vi "Module Template SM.vi"(8 "error in (no error)":errorcluster, 11 "Module_Refs":T1={"ModuleName"=enum."Controller", "Queue"=refnum, "user event"=refnum, "VI Refnum"=refnum, "ShowFP"=FALSE, "StatesTracking Enabled"=FALSE}) -> (0 "error out":errorcluster)   [LabVIEW 2021, in "Module Template.lvlib"]
doc: "Main Module Template of the architecture. Use this as a template to integrate new independent processes into your application."
uses:
  Module Template.lvlib
  Typedefs/Module References.ctl
  Typedefs/Enum_Module_Name.ctl
  Typedefs/Message.ctl
  Typedefs/State Machine Data.ctl
  Typedefs/Config.ctl
  Typedefs/Application Configuration.ctl
  Module Template Configuraton Extractor API.vi
  Configuration/Configuration.lvlib
  Architecture.lvlib
panel:
  in  "Stop App":bool
  out "Message":string
  in  "Stop Module":bool
  # "#Architecture\n\nPlace inside this box all visible data."
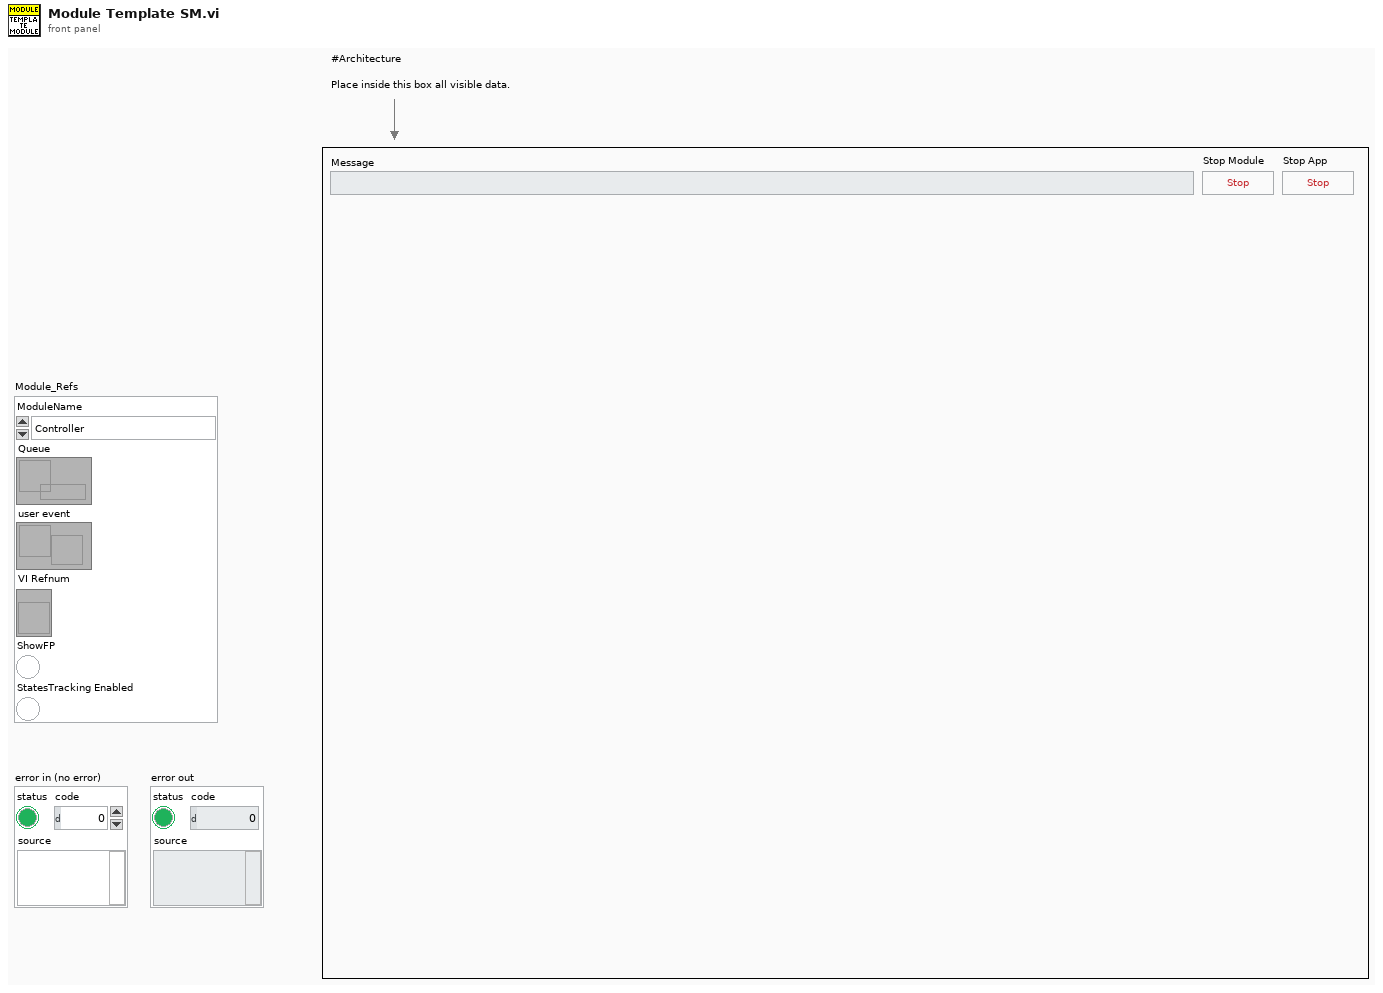
[diagram p1: front panel]
types:
  T1 = typedef "Architecture.lvlib/Module References.ctl" = cluster{"ModuleName":T2, "Queue":refnum<queue>, "user event":refnum<user-event>, "VI Refnum":refnum<vi>, "ShowFP":bool, "StatesTracking Enabled":bool}
  T2 = typedef "Configuration.lvlib/Enum_Module_Name.ctl" = enum16{"Configuration", "Error_Handler", "Log", "Database", "Controller"}
  T3 = typedef "Module Template.lvlib/State Machine Data.ctl" = cluster{"Module_Refs":T1, "Response Data":variant, "Module Template Config":T4}
  T4 = typedef "Module Template.lvlib/Config.ctl" = cluster{"Module Enabled":bool}
  T5 = enum32{"Invalid", "Standard", "Closed", "Hidden", "Minimized", "Maximized"}
  T6 = typedef "Error_Manager.lvlib/LogRotate.lvclass/LogData.ctl" = cluster{"error in":errorcluster, "replacements":string[], "Time Stamp":timestamp}
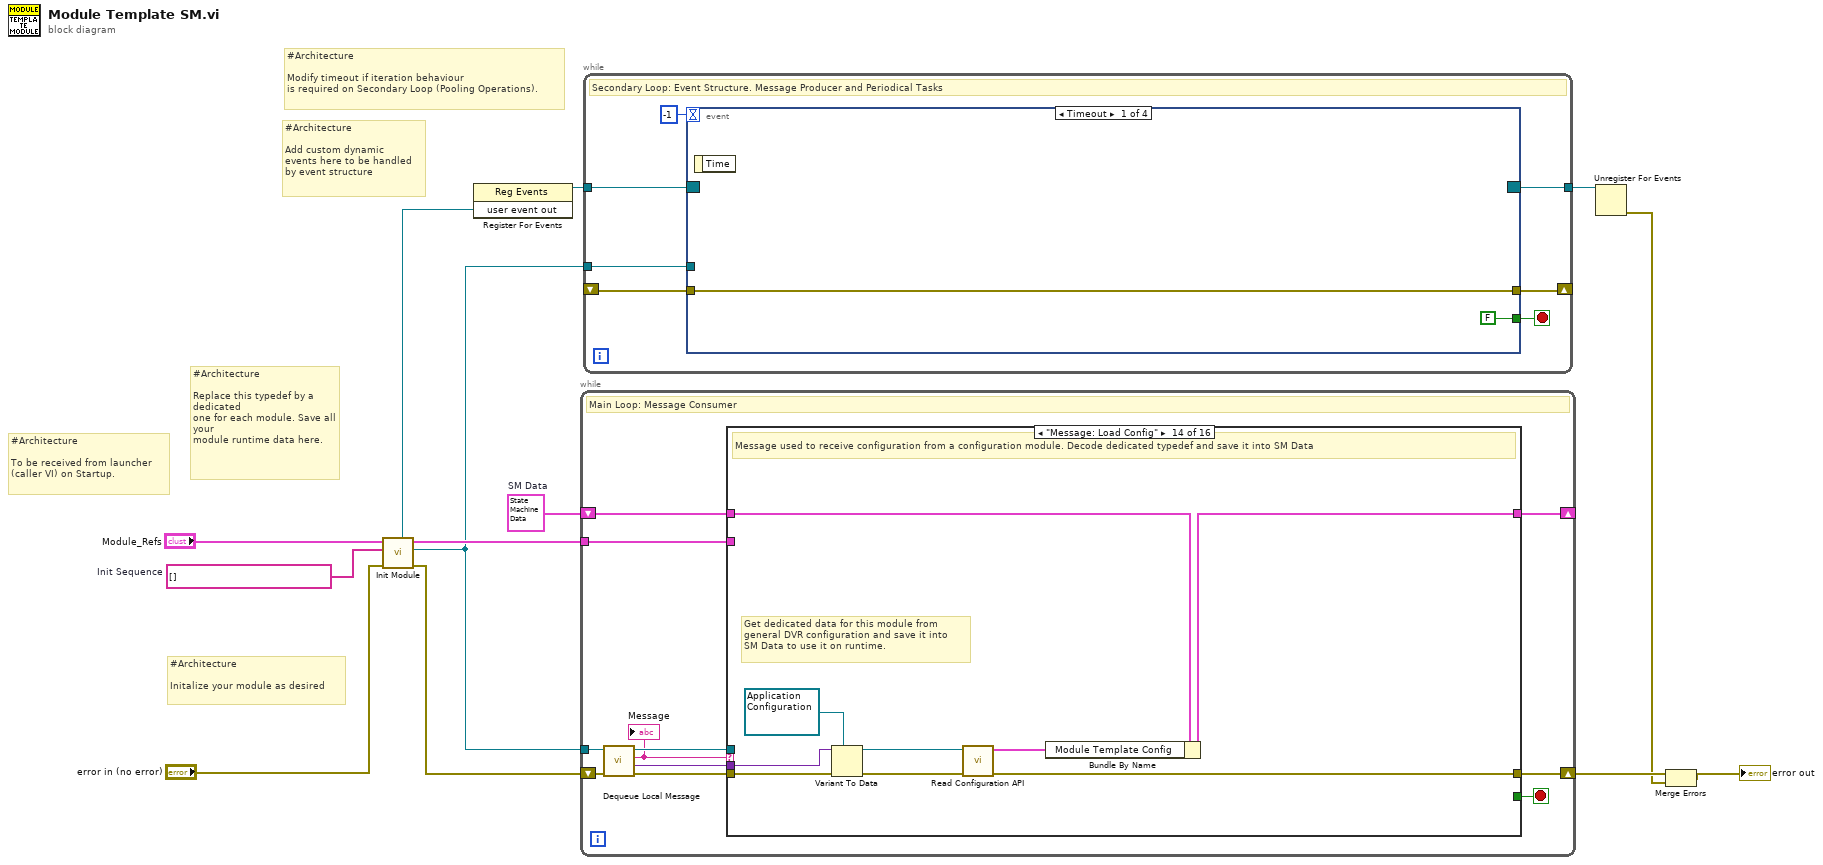
[diagram p0: block diagram]
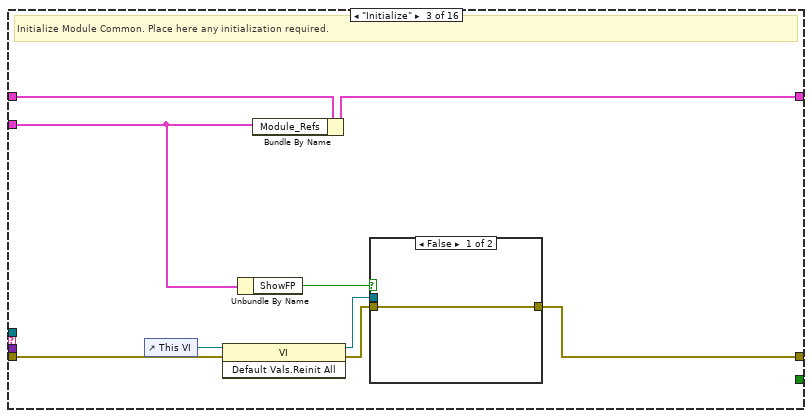
[diagram p4: hidden frame]
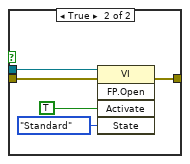
[diagram p5: hidden frame]
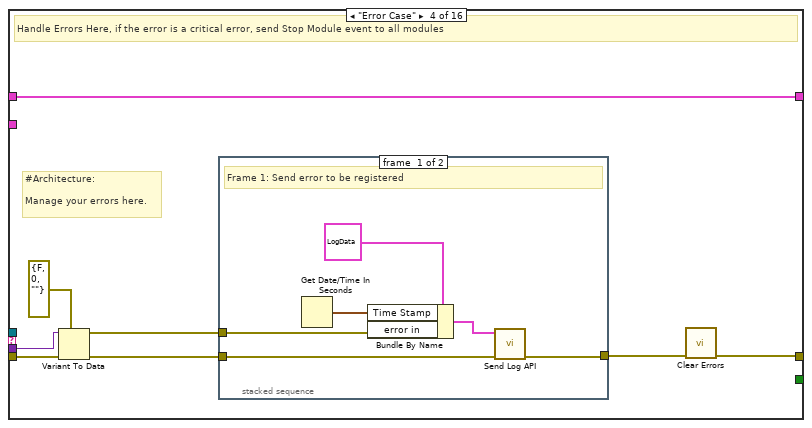
[diagram p6: hidden frame]
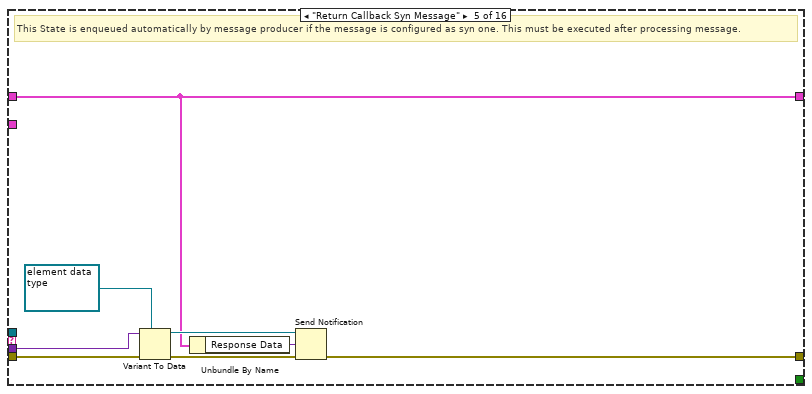
[diagram p9: hidden frame]
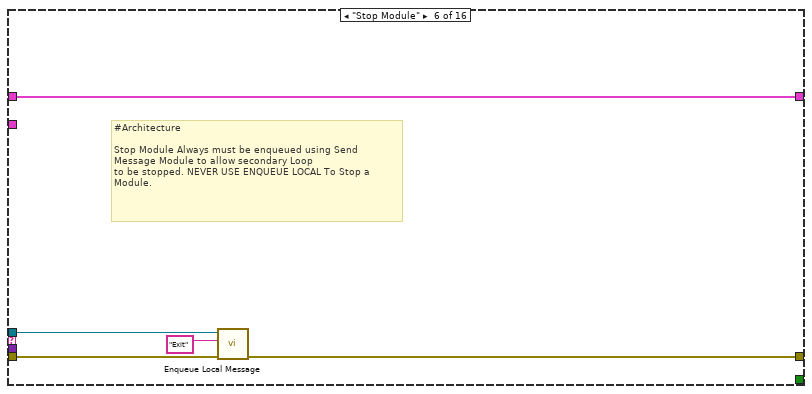
[diagram p10: hidden frame]
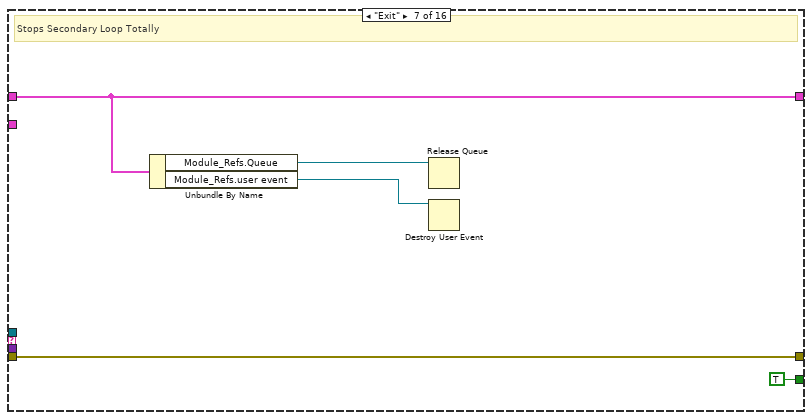
[diagram p11: hidden frame]
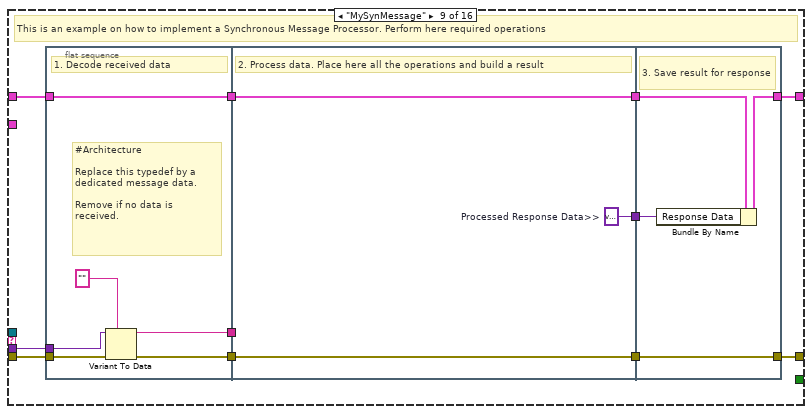
[diagram p13: hidden frame]
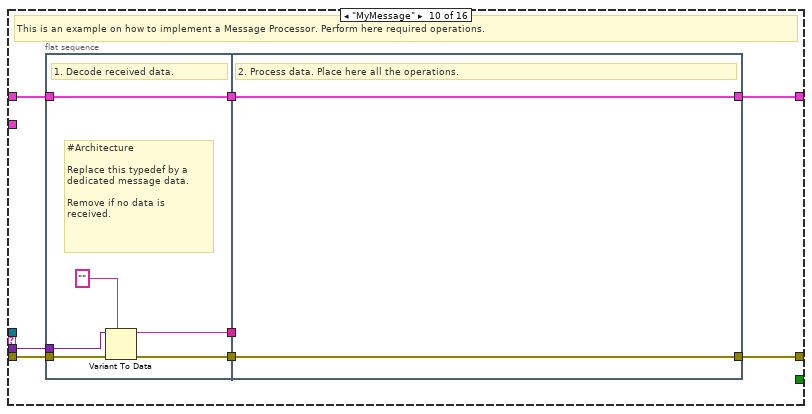
[diagram p14: hidden frame]
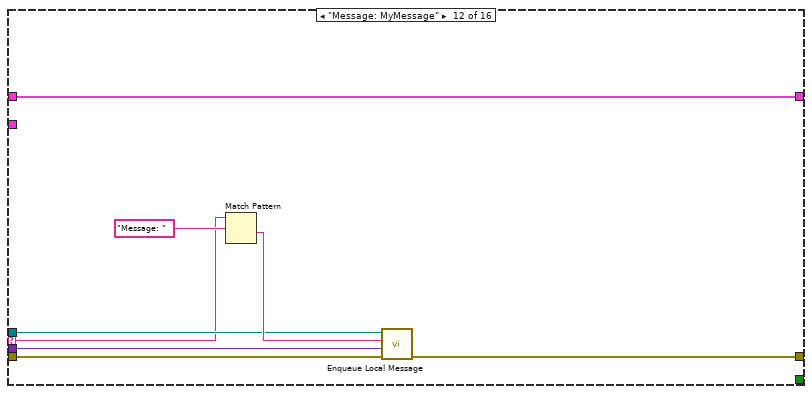
[diagram p16: hidden frame]
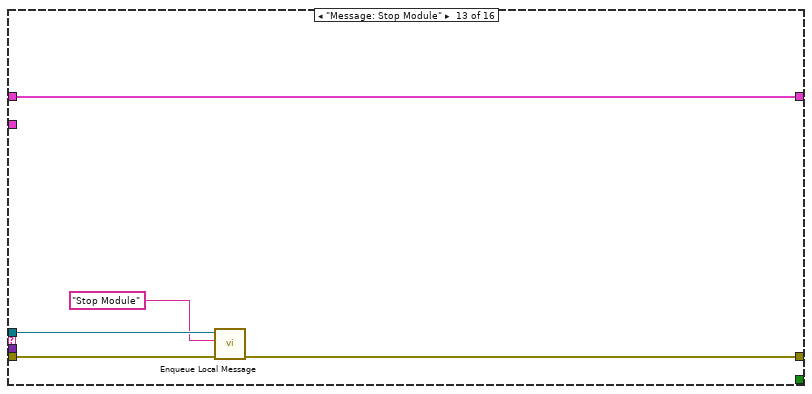
[diagram p17: hidden frame]
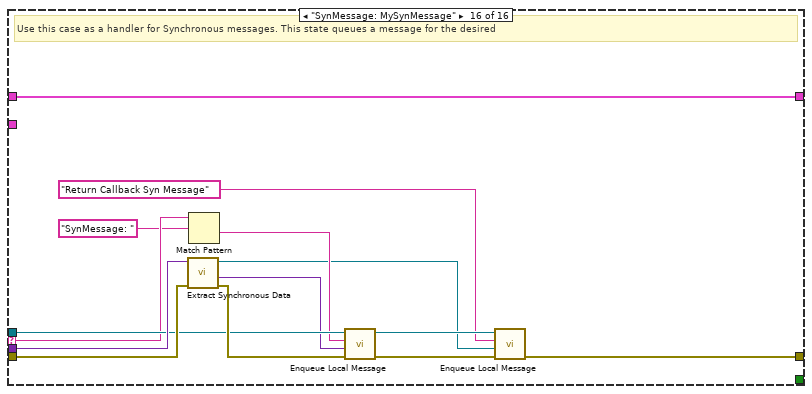
[diagram p19: hidden frame]
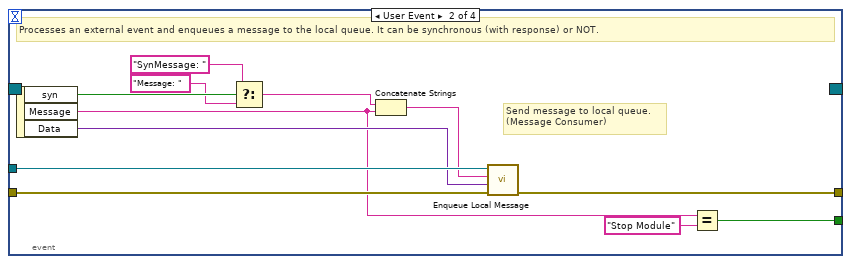
[diagram p20: hidden frame]
diagram:
  w10 = string[] []  # Init Sequence
  w13 = T3 {"Module_Refs"={"ModuleName"=enum."Controller", "Queue"=refnum, "user event"=refnum, "VI Refnum"=refnum, "ShowFP"=FALSE, "StatesTracking Enabled"=FALSE}, "Response Data"=variant, "Module Template Config"={"Module Enabled"=FALSE}}  # SM Data
  # "#Architecture\n\nModify timeout if iteration behaviour \nis required on Secondary Loop (Pooling Operations)."
  # "#Architecture\n\nAdd custom dynamic \nevents here to be handled \nby event structure"
  # "#Architecture\n\nInitalize your module as desired"
  # "#Architecture\n\nTo be received from launcher \n(caller VI) on Startup."
  # "#Architecture\n\nReplace this typedef by a dedicated \none for each module. Save all your \nmodule runtime data here."
  n1 = call "Init Module.vi"("error in (no error)"="error in (no error)", "Init Sequence"=w10, "Module Refs"="Module_Refs") -> ("error out"=w12:errorcluster, "queue out"=w1:refnum<queue>, "Module Refs Out"=w3:T1, "user event out"=w2:refnum<user-event>)  [unwired: 5 in]
  n2 = register-events(w2) -> (reference out=w9:refnum<event-registration>)  [unwired: 2 in, 1 out]
  n3 = while {
    shift-right: [w23] -> _
    shift-left: w13 -> [w24]
    shift-right: [w22] -> w7
    shift-left: w12 -> [w20]
    tunnel: w1 -> [w21]
    tunnel: w3 -> [w14]
    stop <- w15 stop-if-true
    # "Main Loop: Message Consumer"
    n4 = call "Dequeue Local Message.vi"("error in"=w20, "Msg queue in"=w21) -> ("error out"=w19:errorcluster, "Data"=w16:variant, "Message"=w17:string, "queue out"=w18:refnum<queue>)  [unwired: 6 in]
    "Message" <- w17
    n5 = case shown="\"Message: Load Config\"" w17 {
      selector: w17 -> [_ _ _ _ _ _ _ _ _ _ _ w124 _ _ _ w156]
      tunnel: w24 -> [w26 w28 w37 w51 w63 w74 w77 w81 w92 w113 w123 w131 w136 w145 w147 w161]
      tunnel: [w26 w28 w35 w51 w63 w74 w77 w81 w91 w106 w123 w131 w136 w138 w147 w161] -> w23
      tunnel: w19 -> [w25 w27 w36 w50 w69 w73 w79 w80 w85 w109 w122 w128 w135 w144 w146 w160]
      tunnel: [w25 w27 w31 w44 w68 w72 w79 w80 w90 w112 w122 w125 w134 w139 w146 w150] -> w22
      tunnel: w18 -> [_ _ _ _ _ w71 _ _ _ _ _ w126 w133 _ _ w157]
      tunnel: w16 -> [_ _ _ w49 w66 _ _ _ w84 w108 _ w127 _ w143 _ w158]
      tunnel: [_ _ _ _ _ _ TRUE _ _ _ _ _ _ _ _ _] -> w15
      tunnel: w14 -> [_ _ w34 _ _ _ _ _ _ _ _ _ _ _ _ _]
      frame "--------State Machine Arquitechture Operations--------" {
      }
      frame "Idle", Default {
        # "Use this state to make iterations if required."
      }
      frame "Initialize" {
        # "Initialize Module Common. Place here any initialization required."
        n6 = control-ref of="This VI"() -> (w29:refnum<vi>)
        n7 = invoke class="VI" method="Default Vals.Reinit All"(reference=w29, error in=w36) -> (reference out=w32:refnum<vi>, error out=w33:errorcluster)  [unwired: 1 in, 1 out]
        n8 = Unbundle By Name(w34) -> ("ShowFP"=w30:bool)
        n9 = Bundle By Name(cluster=w37, "Module_Refs"=w34) -> (w35:T3)
        n10 = case shown="False" w30 {
          tunnel: w33 -> [w38 w43]
          tunnel: [w38 w42] -> w31
          tunnel: w32 -> [_ w41]
          frame False {
          }
          frame True {
            n11 = invoke class="VI" method="FP.Open"(reference=w41, error in=w43, "Activate"=TRUE ("Activate?"), "State"=T5."Standard") -> (error out=w42:errorcluster)  [unwired: 1 in, 4 out]
          }
        }
      }
      frame "Error Case" {
        # "#Architecture: \n\nManage your errors here."
        # "Handle Errors Here, if the error is a critical error, send Stop Module event to all modules"
        n12 = Variant To Data(error in=w50, type=errorcluster {"status"=FALSE, "code"=0, "source"=""} ("error constant"), Variant=w49) -> (data=w45:errorcluster, error out=w47:errorcluster)
        n13 = stacked-sequence {
          tunnel: w47 -> [w57 w59]
          tunnel: [w56 _] -> w46
          tunnel: w45 -> [w54 w58]
          frame #0 {
            # "Frame 1: Send error to be registered"
            n14 = Get Date/Time In Seconds() -> (seconds since 1Jan1904=w53:timestamp)
            n15 = Bundle By Name(cluster=T6 {"error in"={"status"=FALSE, "code"=0, "source"=""}, "replacements"=[], "Time Stamp"=timestamp(0 s since 1904-01-01)} ("Data"), "Time Stamp"=w53, "error in"=w54) -> (w52:T6)
            n16 = call "Send Log API.vi"("error in (no error)"=w57, "Data"=w52) -> ("error out"=w56:errorcluster)  [unwired: 9 in]
          }
          frame #1 {
            # "Frame 2: Manage your errors here"
            n17 = case shown="No Error" w58 {
              tunnel: [w60 w61] -> _
              tunnel: w59 -> [w60 w61]
              frame No Error {
              }
              frame Error {
                # "#Architecture \n\nPlace here critical errors to be managed \nin the desired way."
              }
            }
          }
        }
        n18 = call <vilib>:"Clear Errors.vi"("error in (no error)"=w46) -> ("error out"=w44:errorcluster)  [unwired: 5 in, 1 out]
      }
      frame "Return Callback Syn Message" {
        # "This State is enqueued automatically by message producer if the message is configured as syn one. This must be executed after processing message."
        n19 = Variant To Data(error in=w69, type=refnum<notifier> refnum ("notifier out"), Variant=w66) -> (data=w64:refnum<notifier>, error out=w67:errorcluster)
        n20 = Unbundle By Name(w63) -> ("Response Data"=w62:variant)
        n21 = Send Notification(notification=w62, notifier=w64, error in (no error)=w67) -> (error out=w68:errorcluster)  [unwired: 1 out]
      }
      frame "Stop Module" {
        # "#Architecture\n\nStop Module Always must be enqueued using Send Message Module to allow secondary Loop\nto be stopped. NEVER USE ENQUEUE LOCAL To Stop a Module."
        n22 = call "Enqueue Local Message.vi"("error in"=w73, "Message"="Exit", "Msg queue in"=w71) -> ("error out"=w72:errorcluster)  [unwired: 7 in, 1 out]
      }
      frame "Exit" {
        # "Stops Secondary Loop Totally"
        n23 = Unbundle By Name(w77) -> ("Module_Refs.Queue"=w76:refnum<queue>, "Module_Refs.user event"=w75:refnum<user-event>)
        n24 = Release Queue(queue=w76) -> ()  [unwired: 2 in, 3 out]
        n25 = Destroy User Event(user event=w75) -> ()  [unwired: 1 in, 1 out]
      }
      frame "--------------State Machine Custom States-------------" {
      }
      frame "MySynMessage" {
        # "This is an example on how to implement a Synchronous Message Processor. Perform here required operations"
        n26 = flat-sequence {
          tunnel: w85 -> [w96]
          tunnel: w92 -> [w98]
          tunnel: [w98] -> w89
          tunnel: [w94] -> w88
          tunnel: w84 -> [w95]
          tunnel: [w93] -> w83
          tunnel: w89 -> [w101]
          tunnel: w88 -> [w100]
          tunnel: [w101] -> w87
          tunnel: [w100] -> w86
          tunnel: w83 -> [_]
          tunnel: [w99] -> w82
          tunnel: [w104] -> w90
          tunnel: [w103] -> w91
          tunnel: w87 -> [w105]
          tunnel: w86 -> [w104]
          tunnel: w82 -> [w102]
          frame #0 {
            # "#Architecture\n\nReplace this typedef by a dedicated message data.\n\nRemove if no data is received."
            # "1. Decode received data"
            n27 = Variant To Data(error in=w96, type="", Variant=w95) -> (data=w93:string, error out=w94:errorcluster)
          }
          frame #1 {
            w99 = variant  # Processed Response Data>>
            # "2. Process data. Place here all the operations and build a result"
          }
          frame #2 {
            # "3. Save result for response"
            n28 = Bundle By Name(cluster=w105, "Response Data"=w102) -> (w103:T3)
          }
        }
      }
      frame "MyMessage" {
        # "This is an example on how to implement a Message Processor. Perform here required operations."
        n29 = flat-sequence {
          tunnel: w109 -> [w117]
          tunnel: w113 -> [w119]
          tunnel: [w119] -> w111
          tunnel: [w115] -> w110
          tunnel: w108 -> [w116]
          tunnel: [w114] -> w107
          tunnel: w111 -> [w120]
          tunnel: w110 -> [w121]
          tunnel: w107 -> [_]
          tunnel: [w121] -> w112
          tunnel: [w120] -> w106
          frame #0 {
            # "#Architecture\n\nReplace this typedef by a dedicated message data.\n\nRemove if no data is received."
            # "1. Decode received data."
            n30 = Variant To Data(error in=w117, type="", Variant=w116) -> (data=w114:string, error out=w115:errorcluster)
          }
          frame #1 {
            # "2. Process data. Place here all the operations."
          }
        }
      }
      frame "--------------Dynamic Events Messages----------------" {
      }
      frame "Message: MyMessage" {
        n31 = Match Pattern(string=w124, regular expression="Message: ") -> (after substring=w129:string)  [unwired: 1 in, 3 out]
        n32 = call "Enqueue Local Message.vi"("error in"=w128, "Data"=w127, "Message"=w129, "Msg queue in"=w126) -> ("error out"=w125:errorcluster)  [unwired: 6 in, 1 out]
      }
      frame "Message: Stop Module" {
        n33 = call "Enqueue Local Message.vi"("error in"=w135, "Message"="Stop Module", "Msg queue in"=w133) -> ("error out"=w134:errorcluster)  [unwired: 7 in, 1 out]
      }
      frame "Message: Load Config" {
        # "Get dedicated data for this module from \ngeneral DVR configuration and save it into \nSM Data to use it on runtime."
        # "Message used to receive configuration from a configuration module. Decode dedicated typedef and save it into SM Data"
        n34 = Variant To Data(error in=w144, type=refnum<data-value> refnum ("data value reference"), Variant=w143) -> (data=w141:refnum<data-value>, error out=w140:errorcluster)
        n35 = call-poly "Read Configuration API.vi"("error constant"=w140, "General Config DVR In"=w141) -> ("error out"=w139:errorcluster, "Module Template Config"=w137:T4)  [unwired: 8 in]
        n36 = Bundle By Name(cluster=w145, "Module Template Config"=w137) -> (w138:T3)
      }
      frame "------------Synchronous Event Messages--------------" {
      }
      frame "SynMessage: MySynMessage" {
        # "Use this case as a handler for Synchronous messages. This state queues a message for the desired"
        n37 = call "Extract Synchronous Data.vi"("error in 2"=w160, "Variant"=w158) -> ("error in"=w159:errorcluster, "Data Out"=w153:variant, "notifier out"=w148:refnum<notifier>)  [unwired: 7 in]
        n38 = Match Pattern(string=w156, regular expression="SynMessage: ") -> (after substring=w154:string)  [unwired: 1 in, 3 out]
        n39 = call "Enqueue Local Message.vi"("error in"=w159, "Data"=w153, "Message"=w154, "Msg queue in"=w157) -> ("error out"=w152:errorcluster, "queue out"=w151:refnum<queue>)  [unwired: 6 in]
        n40 = call "Enqueue Local Message.vi"("error in"=w152, "Data"=w148, "Message"="Return Callback Syn Message", "Msg queue in"=w151) -> ("error out"=w150:errorcluster)  [unwired: 6 in, 1 out]
      }
    }
  }
  n41 = while {
    tunnel: w9 -> [w168]
    tunnel: w1 -> [w165]
    tunnel: [w164] -> w8
    shift-right: [w162] -> _
    shift-left: _ -> [w163]
    stop <- w166 stop-if-true
    # "Secondary Loop: Event Structure. Message Producer and Periodical Tasks"
    n42 = event shown="[0] Timeout" {
      selector: w168 -> [_ _ _ _]
      dyn-events: [_ _ _ _] -> w164
      timeout: -1 -> [_ _ _ _]
      tunnel: [FALSE w177 TRUE _] -> w166
      tunnel: w165 -> [_ w182 w184 _]
      tunnel: w163 -> [w169 w181 w187 w189]
      tunnel: [w169 w180 w185 w188] -> w162
      event Timeout {
        n43 = event-data() -> ()  [unwired: 1 in, 1 out]
      }
      event User Event {
        # "Send message to local queue. \n(Message Consumer)"
        # "Processes an external event and enqueues a message to the local queue. It can be synchronous (with response) or NOT."
        n44 = event-data() -> ("syn"=w174:bool, "Message"=w176:string, "Data"=w179:variant)  [unwired: 1 in]
        n45 = Select(t="SynMessage: " ("string"), s=w174, f="Message: " ("string")) -> (s? t:f=w171:string)
        n46 = Concatenate Strings(w171, w176) -> (w178:string)
        n47 = call "Enqueue Local Message.vi"("error in"=w181, "Data"=w179, "Message"=w178, "Msg queue in"=w182) -> ("error out"=w180:errorcluster)  [unwired: 6 in, 1 out]
        n48 = Equal?(x=w176, y="Stop Module") -> (x = y?=w177:bool)
      }
      event "Stop Module": Value Change {
        n49 = event-data() -> ()  [unwired: 1 in, 1 out]
        n50 = call "Enqueue Local Message.vi"("error in"=w187, "Message"="Stop Module", "Msg queue in"=w184) -> ("error out"=w185:errorcluster)  [unwired: 7 in, 1 out]
      }
      event "Stop App": Value Change {
        w191 = TRUE  # All Modules
        # "Send Stop To All Modules"
        n51 = event-data() -> ()  [unwired: 1 in, 1 out]
        n52 = call "Send Message Modules.vi"("All Modules"=w191, "Error In"=w189, "Message"="Stop Module") -> ("error in (no error)"=w188:errorcluster)  [unwired: 8 in]
      }
    }
  }
  n53 = Unregister For Events(event registration refnum=w8) -> (error out=w6:errorcluster)  [unwired: 1 in]
  n54 = Merge Errors(w7, w6) -> (→"error out":errorcluster)
